vi "IpInputFromUser.vi"(8 "IpStatus (in)":T2[](array[typedef]) {"%rtk" scale=0.0..60.0; "TimePing" scale=0.0..60.0}, 10 "IP":bool, 11 "IP STATUS(in)":T1) -> (0 "IpStatus (out)":T2[](array[typedef]) {"%rtk" scale=0.0..60.0; "TimePing" scale=0.0..60.0}, 3 "IP STATUS(out)":T1, 5 "False":bool)   [LabVIEW 2011]
uses:
  GPS String Capture Software/IP RTK status Indicator.ctl
  ArrayIpAddressesAndReportingCheckbox.ctl
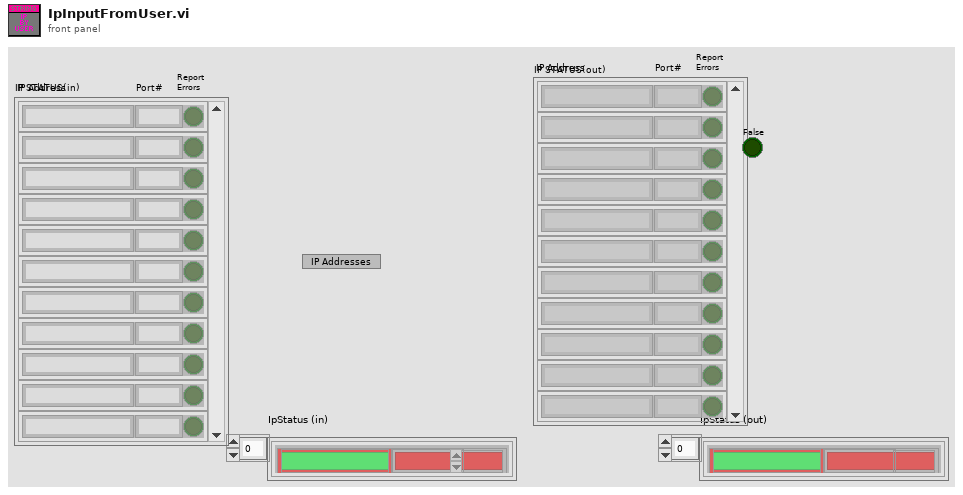
[diagram p1: front panel]
types:
  T1 = typedef "ArrayIpAddressesAndReportingCheckbox.ctl" = cluster{"IpAddress":string, "Report Errors":bool, "IpAddress 2":string}[]
  T2 = typedef "IP RTK status Indicator.ctl" = cluster{"TimePing":dbl, "IP":string, "%rtk":dbl, "Lastrtk":string, "MinLastRTk":dbl, "RTK Count":bool[], "Last Nema Time":dbl, "Last RTK Time":dbl, "Last Ping time":dbl}
  T3 = cluster{"IpAddress":string, "Report Errors":bool, "IpAddress 2":string}
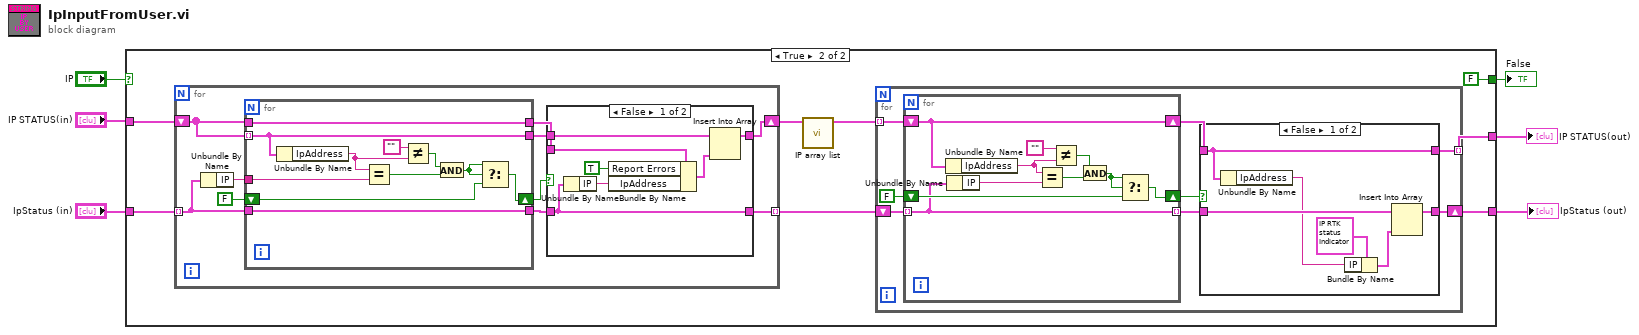
[diagram p0: block diagram]
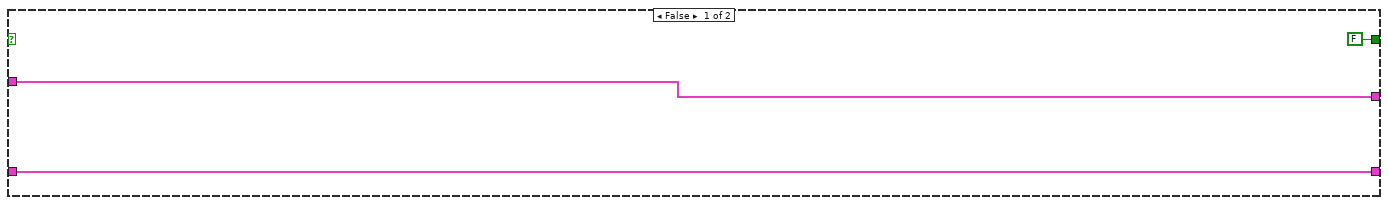
[diagram p2: hidden frame]
diagram:
  n1 = case shown="True" "IP" {
    tunnel: [w9 w17] -> w2
    tunnel: "IP STATUS(in)" -> [w9 w14]
    tunnel: "IpStatus (in)" -> [w8 w15]
    tunnel: [w8 w16] -> w4
    tunnel: [FALSE FALSE] -> w1
    frame False {
    }
    frame True {
      n2 = for {
        tunnel: w15 -> [w25] mode=indexing
        shift-right: [w22] -> w12
        shift-left: w14 -> [w19]
        tunnel: [w20] -> w13 mode=indexing
        n3 = Unbundle By Name(w25) -> ("IP"=w27:string)
        n4 = for {
          tunnel: w27 -> [w47]
          tunnel: w19 -> [w42] mode=indexing
          shift-right: [w45] -> w24
          shift-left: FALSE -> [w46]
          tunnel: w25 -> [w43]
          tunnel: [w43] -> w21
          tunnel: [w42] -> w18
          tunnel: w19 -> [w44]
          tunnel: [w44] -> w23
          n5 = Unbundle By Name(w42) -> ("IpAddress"=w38:string)
          n6 = Equal?(x=w38, y=w47) -> (x = y?=w41:bool)
          n7 = Not Equal?(x="", y=w38) -> (x != y?=w39:bool)
          n8 = And(x=w39, y=w41) -> (x .and. y?=w40:bool)
          n9 = Select(t=w40, s=w40, f=w46) -> (s? t:f=w45:bool)
        }
        n10 = case shown="False" w24 {
          tunnel: w23 -> [w34 w36]
          tunnel: [w33 w36] -> w22
          tunnel: w21 -> [w32 w35]
          tunnel: [w32 w35] -> w20
          tunnel: w18 -> [w31 _]
          frame False {
            n11 = Unbundle By Name(w32) -> ("IP"=w30:string)
            n12 = Bundle By Name(cluster=w31, "Report Errors"=TRUE, "IpAddress"=w30) -> (w29:T3)
            n13 = Insert Into Array(array=w34, new element=w29) -> (w33:T1)  [unwired: 1 in]
          }
          frame True {
          }
        }
      }
      n14 = call "IP array list.vi"("IP STATUS(in)"=w12) -> ("IP STATUS(out)"=w11:T1)  [unwired: 10 in]
      n15 = for {
        tunnel: w11 -> [w54] mode=indexing
        tunnel: [w49] -> w17 mode=indexing
        shift-right: [w48] -> w16
        shift-left: w13 -> [w55]
        n16 = for {
          tunnel: w55 -> [w70] mode=indexing
          shift-right: [w71] -> w52
          shift-left: FALSE -> [w72]
          tunnel: [w70] -> w51 mode=indexing
          shift-right: [w69] -> w50
          shift-left: w54 -> [w69]
          n17 = Unbundle By Name(w69) -> ("IpAddress"=w65:string)
          n18 = Unbundle By Name(w70) -> ("IP"=w73:string)
          n19 = Equal?(x=w65, y=w73) -> (x = y?=w67:bool)
          n20 = Not Equal?(x="", y=w65) -> (x != y?=w66:bool)
          n21 = And(x=w66, y=w67) -> (x .and. y?=w68:bool)
          n22 = Select(t=w68, s=w68, f=w72) -> (s? t:f=w71:bool)
        }
        n23 = case shown="False" w52 {
          tunnel: w51 -> [w60 w62]
          tunnel: w50 -> [w57 w63]
          tunnel: [w57 w63] -> w49
          tunnel: [w61 w62] -> w48
          frame False {
            n24 = Unbundle By Name(w57) -> ("IpAddress"=w56:string)
            n25 = Bundle By Name(cluster=T2 {"TimePing"=0.0, "IP"="", "%rtk"=0.0, "Lastrtk"="", "MinLastRTk"=0.0, "RTK Count"=[], "Last Nema Time"=0.0, "Last RTK Time"=0.0, "Last Ping time"=0.0} ("IP Status"), "IP"=w56) -> (w59:T2)
            n26 = Insert Into Array(array=w60, new element=w59) -> (w61:T2[])  [unwired: 1 in]
          }
          frame True {
          }
        }
      }
    }
  }
  "IpStatus (out)" <- w4
  "IP STATUS(out)" <- w2
  "False" <- w1
